vi "niRFUtil TRC Histogram.vi"(0 "Trace In":T2 format="%.2f", 5 "Max Bin":dbl format="%.2f", 7 "Min Bin":dbl format="%.2f", 9 "Bin Size":dbl format="%.2f", 13 "Measurement Reset? (T)":T1=TRUE) -> (4 "Histogram Out":i32[](array[numeric]))   [LabVIEW 2015, in "niRFUtil.lvlib"]
doc: "(c) Copyright 2006, National Instruments, Inc. This VI may not be duplicated, sold, or distributed without written consent from National Instruments."
uses:
  niRFUtil.lvlib
  Includes/niRFUtil INC Trace.ctl
  Includes/niRFUtil INC Measurement Reset.ctl
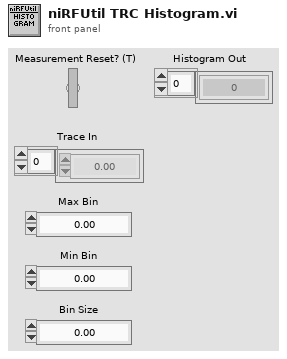
[diagram p1: front panel]
types:
  T1 = typedef "niRFUtil.lvlib/niRFUtil INC Measurement Reset.ctl" = bool
  T2 = typedef "niRFUtil.lvlib/niRFUtil INC Trace.ctl" = sgl[]
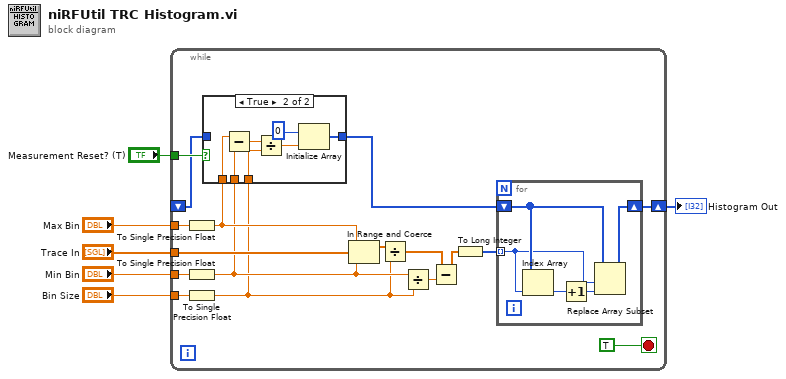
[diagram p0: block diagram]
diagram:
  n1 = while {
    tunnel: "Trace In" -> [w23]
    tunnel: "Min Bin" -> [w14]
    tunnel: "Max Bin" -> [w15]
    tunnel: "Bin Size" -> [w13]
    shift-right: [w22] -> w2
    shift-left: _ -> [w11]
    tunnel: "Measurement Reset? (T)" -> [w16]
    stop <- TRUE stop-if-true
    n2 = To Single Precision Float(number=w15) -> (single precision float=w9:sgl)
    n3 = To Single Precision Float(number=w14) -> (single precision float=w8:sgl)
    n4 = To Single Precision Float(number=w13) -> (single precision float=w7:sgl)
    n5 = case shown="True" w16 {
      tunnel: w9 -> [_ w28]
      tunnel: w8 -> [_ w27]
      tunnel: w7 -> [_ w26]
      tunnel: [w24 w25] -> w12
      tunnel: w11 -> [w24 _]
      frame False {
      }
      frame True {
        n6 = Subtract(x=w28, y=w27) -> (x-y=w30:sgl)
        n7 = Divide(x=w30, y=w26) -> (x/y=w29:sgl)
        n8 = Initialize Array(0 ("Numeric"), w29) -> (w25:i32[])
      }
    }
    n9 = In Range and Coerce(upper limit=w9, x=w23, lower limit=w8) -> (coerced(x)=w21:sgl[])  [unwired: 1 out]
    n10 = Divide(x=w21, y=w7) -> (x/y=w18:sgl[])
    n11 = Divide(x=w8, y=w7) -> (x/y=w19:sgl)
    n12 = Subtract(x=w18, y=w19) -> (x-y=w17:sgl[])
    n13 = To Long Integer(number=w17) -> (32bit integer=w20:i32[])
    n14 = for {
      tunnel: w20 -> [w32] mode=indexing
      shift-right: [w33] -> w22
      shift-left: w12 -> [w34]
      n15 = Index Array(array=w34, index=w32) -> (element=w36:i32)
      n16 = Increment(x=w36) -> (x+1=w35:i32)
      n17 = Replace Array Subset(array=w34, new element=w35, index=w32) -> (w33:i32[])
    }
  }
  "Histogram Out" <- w2
